vi "HEWH Channel Test Labels.vi"(0 "RunTime":bool) -> (3 "MW100 Channel Label":string[](array[string]), 4 "Agilent Cluster Array":T2[](array[typedef]), 6 "Channel List":string)   [LabVIEW 2016]
uses:
  Type Definitions/HEWH Channel Label.ctl
  Type Definitions/HEWH Agilent Cluster.ctl
  <vilib>/Utility/file.llb/Write To Spreadsheet File (string).vi
  <vilib>/Utility/file.llb/Read From Spreadsheet File (string).vi
panel:
  in  "Sensor 5":T1
  in  "Read TC Tree":bool
  out "Description":string="Thermocouple Setup"
  in  "Tab Control":enum32{"Page 1", "Page 2"}(tab)
  out "Agilent TC Locations":string[][](array[string])
  in  "Read":bool
  in  "Write":bool
  in  "Sensor 4":T1
  in  "Read None":bool
  in  "Sensor 3":T1
  in  "Read All":bool
  in  "Complete":bool
  in  "Panel 3":T1[][](array[typedef])=[[{"Label"="TC Cond1 - IN", "Chan"="301", "Rec"=TRUE}, {"Label"="TC Cond2", "Chan"="302", "Rec"=TRUE}, {"Label"="TC Cond3", "Chan"="303", "Rec"=TRUE}, {"Label"="TC Cond4", "Chan"="304", "Rec"=TRUE}, {"Label"="TC Cond5", "Chan"="305", "Rec"=TRUE}, {"Label"="TC Cond6", "Chan"="306", "Rec"=TRUE}], [{"Label"="TC Cond7", "Chan"="307", "Rec"=TRUE}, {"Label"="TC Cond8", "Chan"="308", "Rec"=TRUE}, {"Label"="TC Cond9", "Chan"="309", "Rec"=TRUE}, {"Label"="TC Cond10", "Chan"="310", "Rec"=TRUE}, {"Label"="TC Cond11", "Chan"="311", "Rec"=TRUE}, {"Label"="TC Cond12 - OUT", "Chan"="312", "Rec"=TRUE}], [{"Label"="TC Xtra 4", "Chan"="313", "Rec"=TRUE}, {"Label"="TC Xtra 5", "Chan"="314", "Rec"=TRUE}, {"Label"="TC Xtra 6", "Chan"="315", "Rec"=TRUE}, {"Label"="TC Xtra 7", "Chan"="316", "Rec"=TRUE}, {"Label"="TC Xtra 8", "Chan"="105", "Rec"=TRUE}, {"Label"="TC Xtra 9", "Chan"="106", "Rec"=TRUE}]]
  in  "Panel 2":T1[][](array[typedef])=[[{"Label"="TC Dry/W bulb 1", "Chan"="201", "Rec"=TRUE}, {"Label"="TC Dry/W bulb 2", "Chan"="202", "Rec"=TRUE}, {"Label"="TC Dry/W bulb 3", "Chan"="203", "Rec"=TRUE}, {"Label"="TC Dry/W bulb 4", "Chan"="204", "Rec"=TRUE}, {"Label"="TC Tsuction", "Chan"="205", "Rec"=TRUE}, {"Label"="TC Tdis", "Chan"="206", "Rec"=TRUE}], [{"Label"="TC Tret", "Chan"="207", "Rec"=TRUE}, {"Label"="TC Controls 1", "Chan"="208", "Rec"=TRUE}, {"Label"="TC Controls 2", "Chan"="209", "Rec"=TRUE}, {"Label"="TC Controls 3", "Chan"="210", "Rec"=TRUE}, {"Label"="TC Controls 4", "Chan"="211", "Rec"=TRUE}, {"Label"="TC Controls 5", "Chan"="212", "Rec"=TRUE}], [{"Label"="TC Shadow T1", "Chan"="213", "Rec"=TRUE}, {"Label"="TC Shadow T2", "Chan"="214", "Rec"=TRUE}, {"Label"="TC Shadow T3", "Chan"="215", "Rec"=TRUE}, {"Label"="TC Shadow T4", "Chan"="216", "Rec"=TRUE}, {"Label"="TC Shadow T5", "Chan"="107", "Rec"=TRUE}, {"Label"="TC Shadow T6", "Chan"="108", "Rec"=TRUE}]]
  in  "Panel 1":T1[][](array[typedef])=[[{"Label"="TC Tree 1 - TOP", "Chan"="", "Rec"=TRUE}, {"Label"="TC Tree 2", "Chan"="", "Rec"=TRUE}, {"Label"="TC Tree 3", "Chan"="", "Rec"=TRUE}, {"Label"="TC Tree 4", "Chan"="", "Rec"=TRUE}, {"Label"="TC Tree 5", "Chan"="", "Rec"=TRUE}, {"Label"="TC Tree 6 - BOT", "Chan"="", "Rec"=TRUE}], [{"Label"="TC Shell 1", "Chan"="", "Rec"=TRUE}, {"Label"="TC Shell 2", "Chan"="", "Rec"=TRUE}, {"Label"="TC Shell 3", "Chan"="", "Rec"=TRUE}, {"Label"="TC Shell 4", "Chan"="", "Rec"=TRUE}, {"Label"="TC Evap1 - IN", "Chan"="111", "Rec"=TRUE}, {"Label"="TC Evap2", "Chan"="112", "Rec"=TRUE}], [{"Label"="TC Evap3", "Chan"="113", "Rec"=TRUE}, {"Label"="TC Evap4", "Chan"="114", "Rec"=TRUE}, {"Label"="TC Evap5 - OUT", "Chan"="115", "Rec"=TRUE}, {"Label"="TC Xtra 1", "Chan"="116", "Rec"=TRUE}, {"Label"="TC Xtra 2", "Chan"="109", "Rec"=TRUE}, {"Label"="TC Xtra 3", "Chan"="1100", "Rec"=TRUE}]]
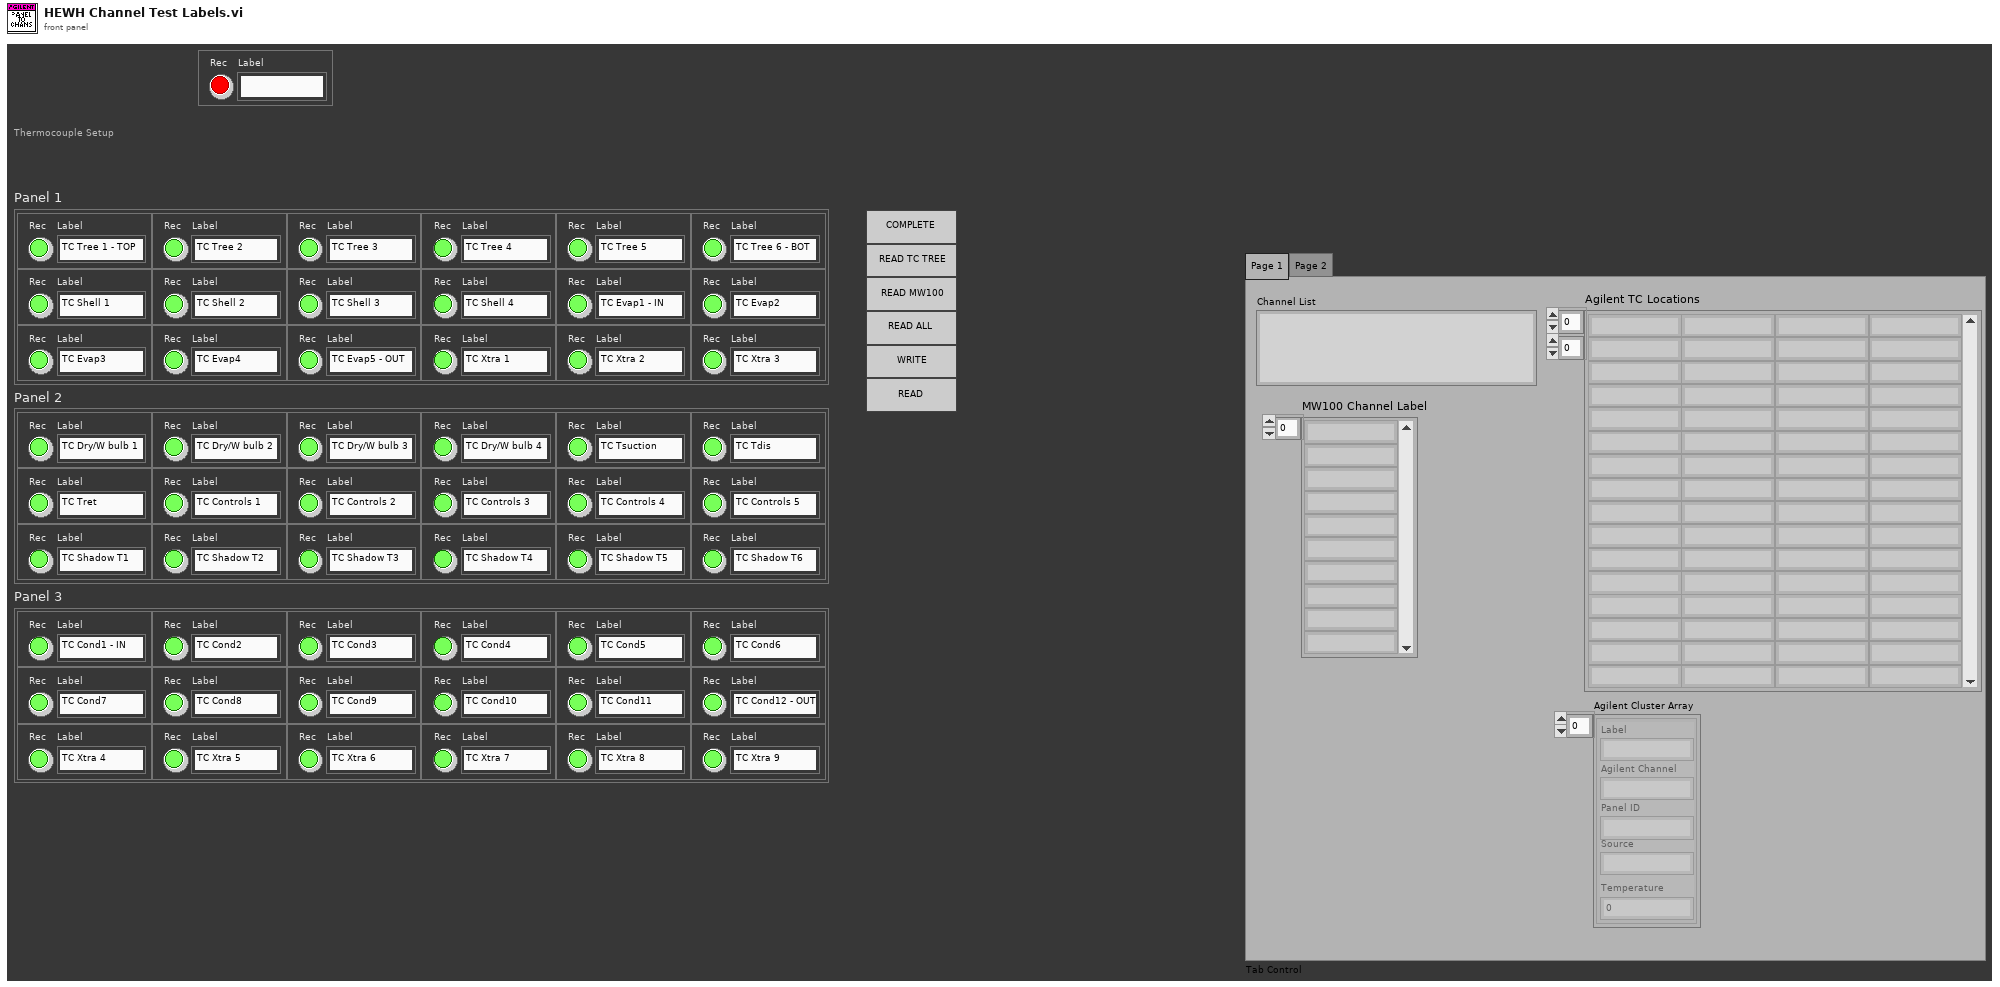
[diagram p1: front panel]
types:
  T1 = typedef "HEWH Channel Label.ctl" = cluster{"Label":string, "Chan":string, "Rec":bool}
  T2 = typedef "HEWH Agilent Cluster.ctl" = cluster{"Label":string, "Agilent Channel":string, "Panel ID":string, "Source":string, "Temperature":dbl}
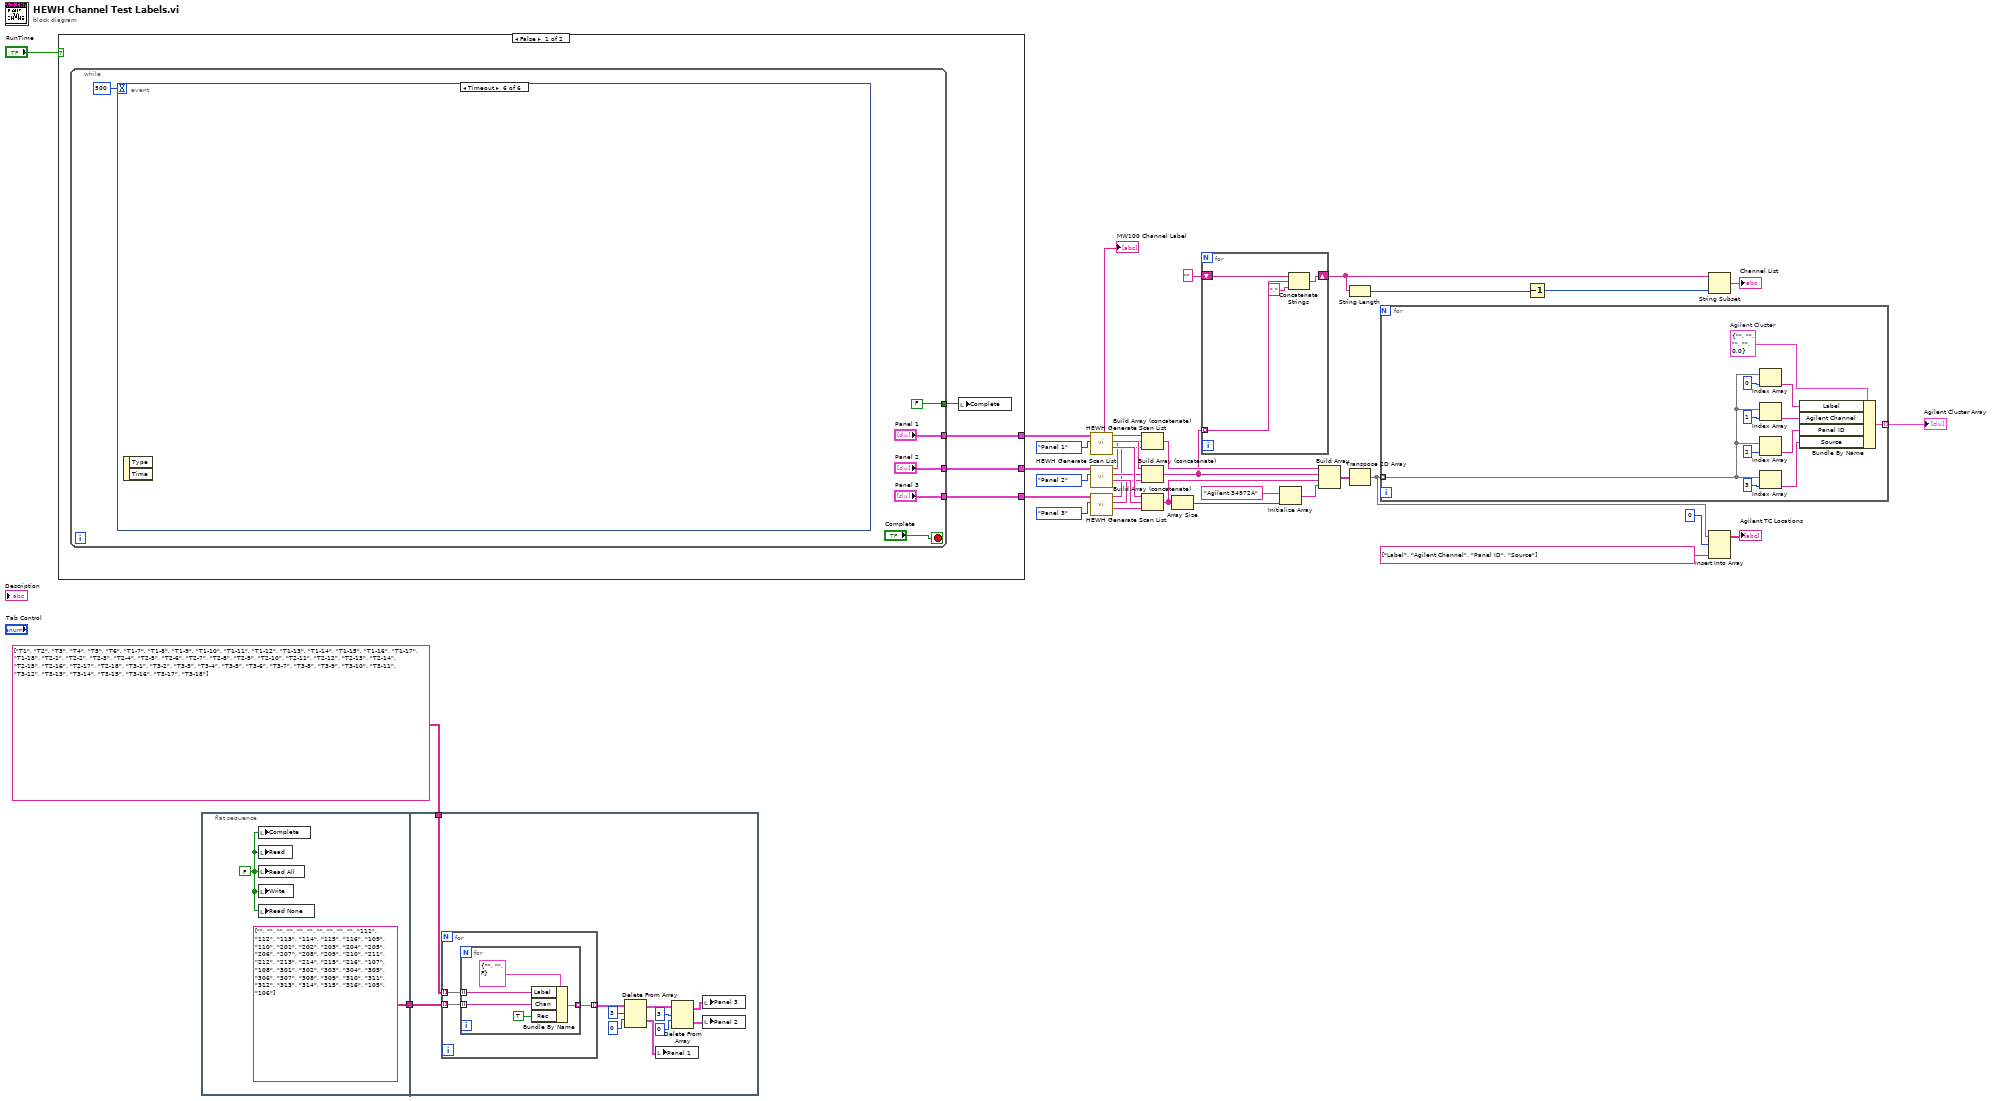
[diagram p0: block diagram]
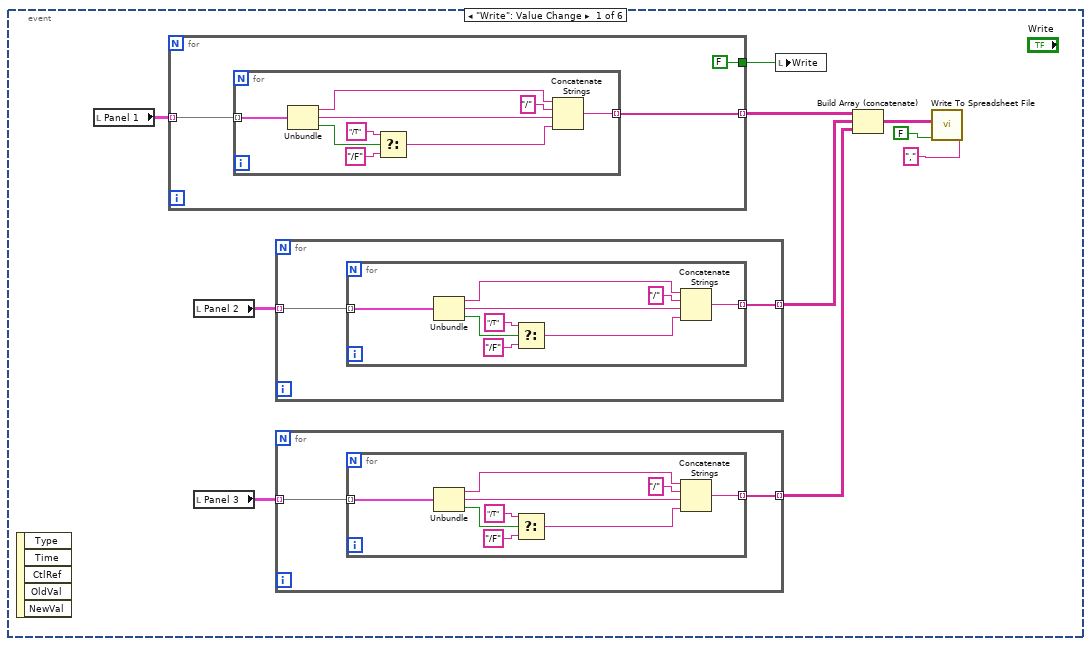
[diagram p2: hidden frame]
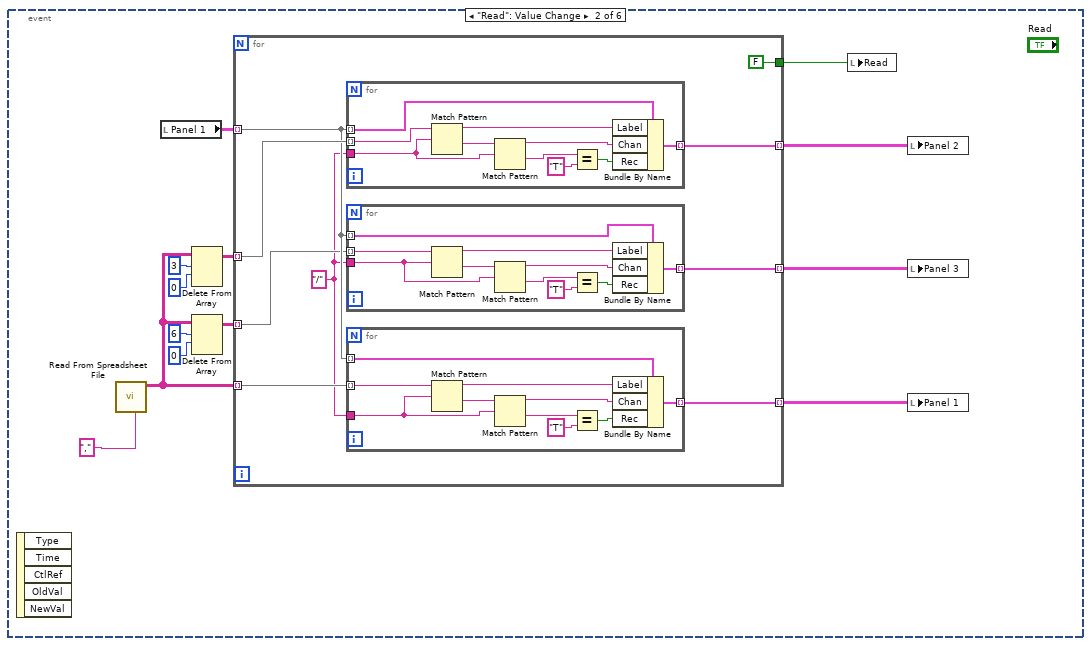
[diagram p3: hidden frame]
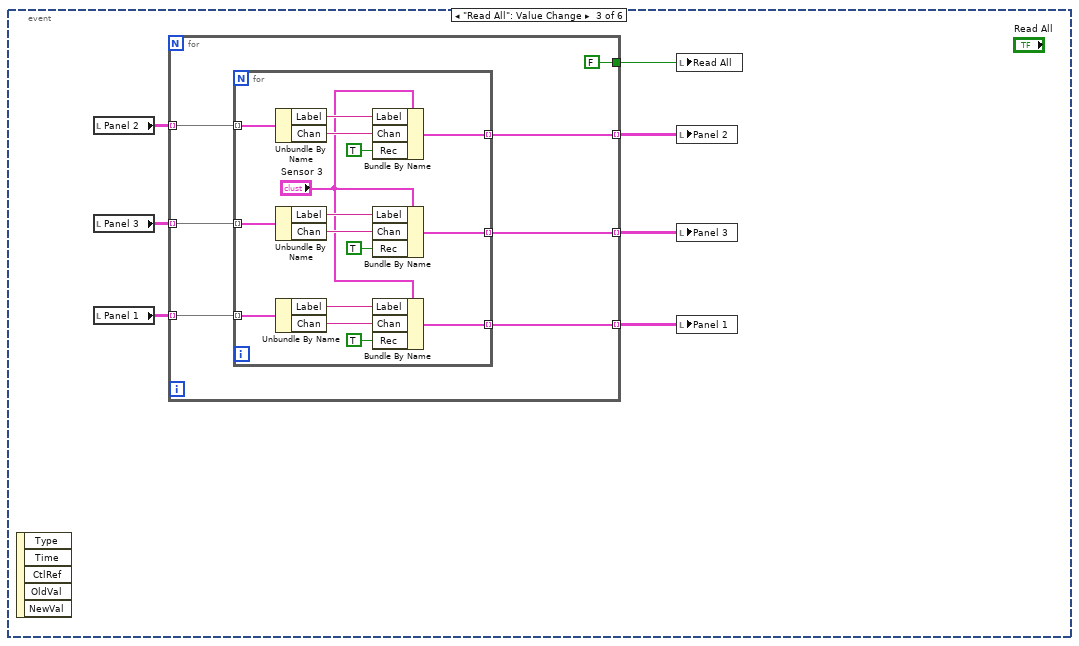
[diagram p4: hidden frame]
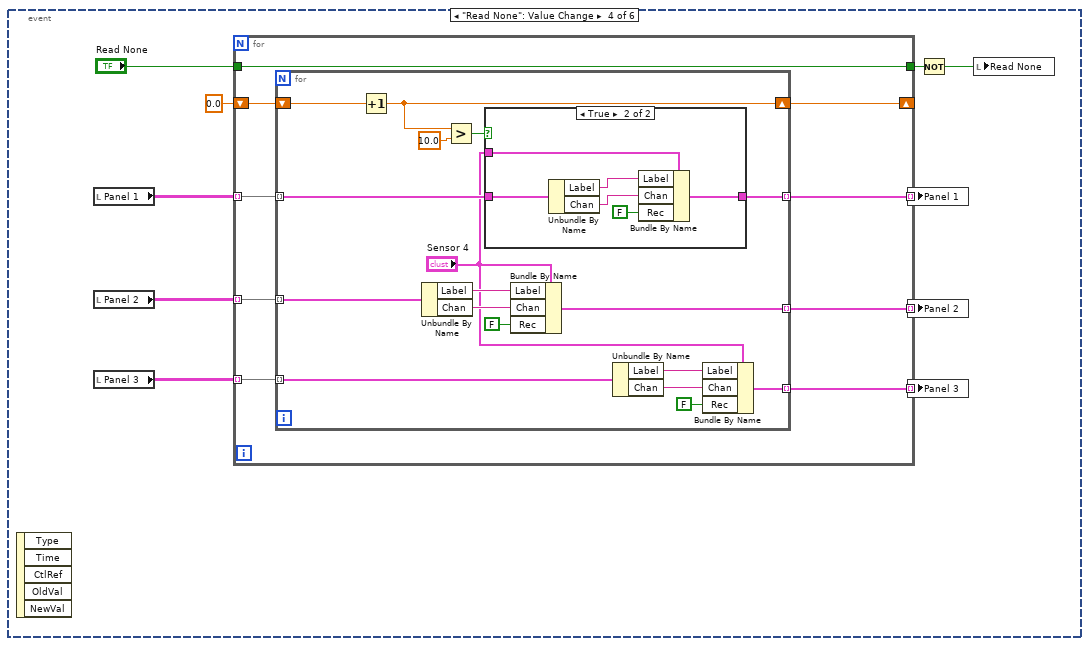
[diagram p5: hidden frame]
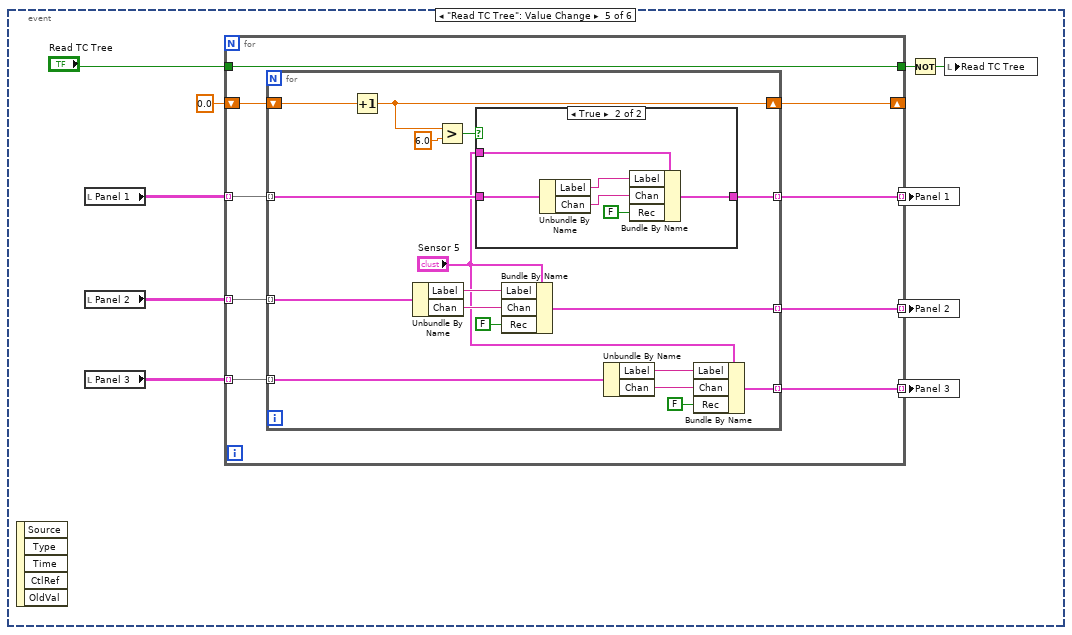
[diagram p7: hidden frame]
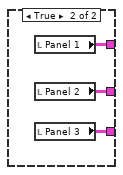
[diagram p9: hidden frame]
diagram:
  n1 = case shown="False" "RunTime" {
    tunnel: [w40 w261] -> w36
    tunnel: [w38 w260] -> w23
    tunnel: [w37 w259] -> w21
    frame False {
      n2 = while {
        tunnel: ["Panel 1"] -> w40
        tunnel: ["Panel 2"] -> w38
        tunnel: ["Panel 3"] -> w37
        tunnel: [FALSE ("Read None")] -> w39
        stop <- "Complete" stop-if-true
        n3 = event shown="[5] Timeout" {
          selector: _ -> [_ _ _ _ _ _]
          dyn-events: _ -> [_ _ _ _ _ _]
          timeout: 500 -> [_ _ _ _ _ _]
          event "Write": Value Change {
            n4 = event-data() -> ()  [unwired: 1 in, 5 out]
            n5 = local read "Panel 1"() -> (w55:T1[][])
            n6 = for {
              tunnel: w55 -> [w81] mode=indexing
              tunnel: [FALSE ("Read None")] -> w56
              tunnel: [w79] -> w51 mode=indexing
              n7 = for {
                tunnel: w81 -> [w90] mode=indexing
                tunnel: [w82] -> w79 mode=indexing
                n8 = Unbundle(w90) -> ("Label"=w89:string, "Chan"=w87:string, "Rec"=w84:bool)
                n9 = Select(t="/T" ("string"), s=w84, f="/F" ("string")) -> (s? t:f=w83:string)
                n10 = Concatenate Strings(w89, "/" ("string"), w87, w83) -> (w82:string)
              }
            }
            n11 = local read "Panel 2"() -> (w53:T1[][])
            n12 = local read "Panel 3"() -> (w52:T1[][])
            n13 = for {
              tunnel: w53 -> [w69] mode=indexing
              tunnel: [w68] -> w50 mode=indexing
              n14 = for {
                tunnel: w69 -> [w78] mode=indexing
                tunnel: [w70] -> w68 mode=indexing
                n15 = Unbundle(w78) -> ("Label"=w77:string, "Chan"=w75:string, "Rec"=w72:bool)
                n16 = Select(t="/T" ("string"), s=w72, f="/F" ("string")) -> (s? t:f=w71:string)
                n17 = Concatenate Strings(w77, "/" ("string"), w75, w71) -> (w70:string)
              }
            }
            n18 = for {
              tunnel: w52 -> [w58] mode=indexing
              tunnel: [w57] -> w49 mode=indexing
              n19 = for {
                tunnel: w58 -> [w67] mode=indexing
                tunnel: [w59] -> w57 mode=indexing
                n20 = Unbundle(w67) -> ("Label"=w66:string, "Chan"=w64:string, "Rec"=w61:bool)
                n21 = Select(t="/T" ("string"), s=w61, f="/F" ("string")) -> (s? t:f=w60:string)
                n22 = Concatenate Strings(w66, "/" ("string"), w64, w60) -> (w59:string)
              }
            }
            n23 = local write "Write"(w56) -> ()
            n24 = Build Array (concatenate)(w51, w50, w49) -> (w47:string[][])
            n25 = call-poly <vilib>:"Write To Spreadsheet File.vi"("delimiter (\\t)"="," ("delimiter (\\t)"), "append to file? (new file:F)"=FALSE ("Keep Refnum Open"), "2D data"=w47) -> ()  [unwired: 5 in, 1 out]
          }
          event "Read": Value Change {
            n26 = event-data() -> ()  [unwired: 1 in, 5 out]
            n27 = call-poly <vilib>:"Read From Spreadsheet File.vi"("delimiter (\\t)"="," ("delimiter (\\t)")) -> ("all rows"=w97:string[][])  [unwired: 6 in, 4 out]
            n28 = local read "Panel 1"() -> (w93:T1[][])
            n29 = Delete From Array(array=w97, length=3, index (row)=0) -> (array with subset deleted=w98:string[][])  [unwired: 1 in, 1 out]
            n30 = Delete From Array(array=w97, length=6, index (row)=0) -> (array with subset deleted=w99:string[][])  [unwired: 1 in, 1 out]
            n31 = for {
              tunnel: w93 -> [w107] mode=indexing
              tunnel: w97 -> [w112] mode=indexing
              tunnel: [w111] -> w96 mode=indexing
              tunnel: w98 -> [w110] mode=indexing
              tunnel: w99 -> [w106] mode=indexing
              tunnel: [w109] -> w95 mode=indexing
              tunnel: [w108] -> w94 mode=indexing
              tunnel: [FALSE ("Read")] -> w92
              w105 = "/" ("regular expression")
              n32 = for {
                tunnel: w107 -> [w131] mode=indexing
                tunnel: w110 -> [w132] mode=indexing
                tunnel: [w129] -> w109 mode=indexing
                tunnel: w105 -> [w123]
                n33 = Match Pattern(string=w132, regular expression=w123) -> (before substring=w130:string, after substring=w128:string)  [unwired: 1 in, 2 out]
                n34 = Match Pattern(string=w128, regular expression=w123) -> (before substring=w127:string, after substring=w126:string)  [unwired: 1 in, 2 out]
                n35 = Equal?(x=w126, y="T") -> (x = y?=w124:bool)
                n36 = Bundle By Name(cluster=w131, "Label"=w130, "Chan"=w127, "Rec"=w124) -> (w129:T1)
              }
              n37 = for {
                tunnel: w107 -> [w121] mode=indexing
                tunnel: w106 -> [w122] mode=indexing
                tunnel: [w119] -> w108 mode=indexing
                tunnel: w105 -> [w113]
                n38 = Match Pattern(string=w122, regular expression=w113) -> (before substring=w120:string, after substring=w118:string)  [unwired: 1 in, 2 out]
                n39 = Match Pattern(string=w118, regular expression=w113) -> (before substring=w117:string, after substring=w116:string)  [unwired: 1 in, 2 out]
                n40 = Equal?(x=w116, y="T") -> (x = y?=w114:bool)
                n41 = Bundle By Name(cluster=w121, "Label"=w120, "Chan"=w117, "Rec"=w114) -> (w119:T1)
              }
              n42 = for {
                tunnel: w107 -> [w141] mode=indexing
                tunnel: w112 -> [w142] mode=indexing
                tunnel: [w139] -> w111 mode=indexing
                tunnel: w105 -> [w133]
                n43 = Match Pattern(string=w142, regular expression=w133) -> (before substring=w140:string, after substring=w138:string)  [unwired: 1 in, 2 out]
                n44 = Match Pattern(string=w138, regular expression=w133) -> (before substring=w137:string, after substring=w136:string)  [unwired: 1 in, 2 out]
                n45 = Equal?(x=w136, y="T") -> (x = y?=w134:bool)
                n46 = Bundle By Name(cluster=w141, "Label"=w140, "Chan"=w137, "Rec"=w134) -> (w139:T1)
              }
            }
            n47 = local write "Read"(w92) -> ()
            n48 = local write "Panel 2"(w95) -> ()
            n49 = local write "Panel 3"(w94) -> ()
            n50 = local write "Panel 1"(w96) -> ()
          }
          event "Read All": Value Change {
            n51 = event-data() -> ()  [unwired: 1 in, 5 out]
            n52 = local read "Panel 2"() -> (w146:T1[][])
            n53 = local read "Panel 3"() -> (w145:T1[][])
            n54 = local read "Panel 1"() -> (w149:T1[][])
            n55 = for {
              tunnel: [w156] -> w148 mode=indexing
              tunnel: w149 -> [w155] mode=indexing
              tunnel: [w154] -> w147 mode=indexing
              tunnel: w146 -> [w153] mode=indexing
              tunnel: w145 -> [w152] mode=indexing
              tunnel: [w151] -> w144 mode=indexing
              tunnel: [FALSE ("Read None")] -> w143
              n56 = for {
                tunnel: [w172] -> w156 mode=indexing
                tunnel: w155 -> [w170] mode=indexing
                tunnel: [w164] -> w154 mode=indexing
                tunnel: w153 -> [w163] mode=indexing
                tunnel: w152 -> [w159] mode=indexing
                tunnel: [w158] -> w151 mode=indexing
                n57 = Unbundle By Name(w163) -> ("Label"=w166:string, "Chan"=w167:string)
                n58 = Unbundle By Name(w159) -> ("Label"=w161:string, "Chan"=w160:string)
                n59 = Unbundle By Name(w170) -> ("Label"=w169:string, "Chan"=w168:string)
                n60 = Bundle By Name(cluster="Sensor 3", "Label"=w166, "Chan"=w167, "Rec"=TRUE) -> (w164:T1)
                n61 = Bundle By Name(cluster="Sensor 3", "Label"=w161, "Chan"=w160, "Rec"=TRUE) -> (w158:T1)
                n62 = Bundle By Name(cluster="Sensor 3", "Label"=w169, "Chan"=w168, "Rec"=TRUE) -> (w172:T1)
              }
            }
            n63 = local write "Read All"(w143) -> ()
            n64 = local write "Panel 2"(w147) -> ()
            n65 = local write "Panel 3"(w144) -> ()
            n66 = local write "Panel 1"(w148) -> ()
          }
          event "Read None": Value Change {
            n67 = event-data() -> ()  [unwired: 1 in, 5 out]
            n68 = local read "Panel 1"() -> (w182:T1[][])
            n69 = local read "Panel 2"() -> (w179:T1[][])
            n70 = local read "Panel 3"() -> (w178:T1[][])
            n71 = for {
              tunnel: [w191] -> w181 mode=indexing
              tunnel: w182 -> [w190] mode=indexing
              tunnel: [w189] -> w180 mode=indexing
              tunnel: w179 -> [w188] mode=indexing
              tunnel: w178 -> [w187] mode=indexing
              tunnel: [w186] -> w177 mode=indexing
              tunnel: [w185] -> w175
              tunnel: "Read None" -> [w185]
              shift-right: [w183] -> _
              shift-left: 0.0 -> [w184]
              n72 = for {
                tunnel: [w208] -> w191 mode=indexing
                tunnel: w190 -> [w207] mode=indexing
                tunnel: [w203] -> w189 mode=indexing
                tunnel: w188 -> [w202] mode=indexing
                tunnel: w187 -> [w198] mode=indexing
                tunnel: [w197] -> w186 mode=indexing
                shift-right: [w194] -> w183
                shift-left: w184 -> [w195]
                n73 = Increment(x=w195) -> (x+1=w194:dbl)
                n74 = Unbundle By Name(w202) -> ("Label"=w205:string, "Chan"=w206:string)
                n75 = Greater?(x=w194, y=10.0) -> (0:w192:bool)
                n76 = case shown="True" w192 {
                  tunnel: [w209 w215] -> w208
                  tunnel: w207 -> [w209 w213]
                  tunnel: "Sensor 4" -> [_ w210]
                  frame False {
                  }
                  frame True {
                    n77 = Unbundle By Name(w213) -> ("Label"=w212:string, "Chan"=w211:string)
                    n78 = Bundle By Name(cluster=w210, "Label"=w212, "Chan"=w211, "Rec"=FALSE) -> (w215:T1)
                  }
                }
                n79 = Bundle By Name(cluster="Sensor 4", "Label"=w205, "Chan"=w206, "Rec"=FALSE) -> (w203:T1)
                n80 = Unbundle By Name(w198) -> ("Label"=w200:string, "Chan"=w199:string)
                n81 = Bundle By Name(cluster="Sensor 4", "Label"=w200, "Chan"=w199, "Rec"=FALSE) -> (w197:T1)
              }
            }
            n82 = local write "Panel 1"(w181) -> ()
            n83 = local write "Panel 2"(w180) -> ()
            n84 = local write "Panel 3"(w177) -> ()
            n85 = Not(x=w175) -> (.not. x?=w176:bool)
            n86 = local write "Read None"(w176) -> ()
          }
          event "Read TC Tree": Value Change {
            n87 = event-data() -> ()  [unwired: 1 in, 5 out]
            n88 = local read "Panel 1"() -> (w225:T1[][])
            n89 = local read "Panel 2"() -> (w222:T1[][])
            n90 = local read "Panel 3"() -> (w221:T1[][])
            n91 = for {
              tunnel: [w234] -> w224 mode=indexing
              tunnel: w225 -> [w233] mode=indexing
              tunnel: [w232] -> w223 mode=indexing
              tunnel: w222 -> [w231] mode=indexing
              tunnel: w221 -> [w230] mode=indexing
              tunnel: [w229] -> w220 mode=indexing
              tunnel: [w228] -> w219
              tunnel: "Read TC Tree" -> [w228]
              shift-right: [w226] -> _
              shift-left: 0.0 -> [w227]
              n92 = for {
                tunnel: [w251] -> w234 mode=indexing
                tunnel: w233 -> [w250] mode=indexing
                tunnel: [w246] -> w232 mode=indexing
                tunnel: w231 -> [w245] mode=indexing
                tunnel: w230 -> [w241] mode=indexing
                tunnel: [w240] -> w229 mode=indexing
                shift-right: [w237] -> w226
                shift-left: w227 -> [w238]
                n93 = Increment(x=w238) -> (x+1=w237:dbl)
                n94 = Unbundle By Name(w245) -> ("Label"=w248:string, "Chan"=w249:string)
                n95 = Greater?(x=w237, y=6.0) -> (0:w235:bool)
                n96 = case shown="True" w235 {
                  tunnel: [w252 w258] -> w251
                  tunnel: w250 -> [w252 w256]
                  tunnel: "Sensor 5" -> [_ w253]
                  frame False {
                  }
                  frame True {
                    n97 = Unbundle By Name(w256) -> ("Label"=w255:string, "Chan"=w254:string)
                    n98 = Bundle By Name(cluster=w253, "Label"=w255, "Chan"=w254, "Rec"=FALSE) -> (w258:T1)
                  }
                }
                n99 = Bundle By Name(cluster="Sensor 5", "Label"=w248, "Chan"=w249, "Rec"=FALSE) -> (w246:T1)
                n100 = Unbundle By Name(w241) -> ("Label"=w243:string, "Chan"=w242:string)
                n101 = Bundle By Name(cluster="Sensor 5", "Label"=w243, "Chan"=w242, "Rec"=FALSE) -> (w240:T1)
              }
            }
            n102 = local write "Panel 1"(w224) -> ()
            n103 = local write "Panel 2"(w223) -> ()
            n104 = local write "Panel 3"(w220) -> ()
            n105 = Not(x=w219) -> (.not. x?=w216:bool)
            n106 = local write "Read TC Tree"(w216) -> ()
          }
          event Timeout {
            n107 = event-data() -> ()  [unwired: 1 in, 2 out]
          }
        }
      }
      n108 = local write "Complete"(w39) -> ()
    }
    frame True {
      n109 = local read "Panel 1"() -> (w261:T1[][])
      n110 = local read "Panel 2"() -> (w260:T1[][])
      n111 = local read "Panel 3"() -> (w259:T1[][])
    }
  }
  n112 = flat-sequence {
    tunnel: [string[][] [["", "", "", "", "", ""], ["", "", "", "", "111", "112"], ["113", "114", "115", "116", "109", "110"], ["201", "202", "203", "204", "205", "206"], ["207", "208", "209", "210", "211", "212"], ["213", "214", "215", "216", "107", "108"], ["301", "302", "303", "304", "305", "306"], ["307", "308", "309", "310", "311", "312"], ["313", "314", "315", "316", "105", "106"]] ("transposed array")] -> w13
    tunnel: w13 -> [w265]
    tunnel: string[][] [["T1", "T2", "T3", "T4", "T5", "T6"], ["T1-7", "T1-8", "T1-9", "T1-10", "T1-11", "T1-12"], ["T1-13", "T1-14", "T1-15", "T1-16", "T1-17", "T1-18"], ["T2-1", "T2-2", "T2-3", "T2-4", "T2-5", "T2-6"], ["T2-7", "T2-8", "T2-9", "T2-10", "T2-11", "T2-12"], ["T2-13", "T2-14", "T2-15", "T2-16", "T2-17", "T2-18"], ["T3-1", "T3-2", "T3-3", "T3-4", "T3-5", "T3-6"], ["T3-7", "T3-8", "T3-9", "T3-10", "T3-11", "T3-12"], ["T3-13", "T3-14", "T3-15", "T3-16", "T3-17", "T3-18"]] ("Array") -> [w264]
    frame #0 {
      w262 = FALSE ("Read None")
      n113 = local write "Complete"(w262) -> ()
      n114 = local write "Read"(w262) -> ()
      n115 = local write "Read All"(w262) -> ()
      n116 = local write "Write"(w262) -> ()
      n117 = local write "Read None"(w262) -> ()
    }
    frame #1 {
      n118 = for {
        tunnel: [w277] -> w274 mode=indexing
        tunnel: w264 -> [w276] mode=indexing
        tunnel: w265 -> [w275] mode=indexing
        n119 = for {
          tunnel: [w282] -> w277 mode=indexing
          tunnel: w276 -> [w281] mode=indexing
          tunnel: w275 -> [w280] mode=indexing
          n120 = Bundle By Name(cluster=T1 {"Label"="", "Chan"="", "Rec"=FALSE} ("Sensor 2"), "Label"=w281, "Chan"=w280, "Rec"=TRUE) -> (w282:T1)
        }
      }
      n121 = Delete From Array(array=w274, length=3, index (row)=0) -> (deleted portion=w268:T1[][], array with subset deleted=w269:T1[][])  [unwired: 1 in]
      n122 = local write "Panel 1"(w268) -> ()
      n123 = Delete From Array(array=w269, length=3, index (row)=0) -> (deleted portion=w267:T1[][], array with subset deleted=w266:T1[][])  [unwired: 1 in]
      n124 = local write "Panel 3"(w266) -> ()
      n125 = local write "Panel 2"(w267) -> ()
    }
  }
  n126 = call "HEWH Generate Scan List.vi"(10:"Panel"=enum16{"Panel 1", "Panel 2", "Panel 3"}."Panel 1" ("Panel"), 11:"Panel"=w36) -> ("Panel List"=w28:string[], "Channel Number"=w34:string[], "Channel Label"=w35:string[], "MW100 Channel Label"=→"MW100 Channel Label":string[])  [unwired: 6 in]
  n127 = call "HEWH Generate Scan List.vi"(10:"Panel"=enum16{"Panel 1", "Panel 2", "Panel 3"}."Panel 2" ("Panel"), 11:"Panel"=w23) -> ("Panel List"=w19:string[], "Channel Number"=w17:string[], "Channel Label"=w18:string[])  [unwired: 6 in, 1 out]
  n128 = call "HEWH Generate Scan List.vi"(10:"Panel"=enum16{"Panel 1", "Panel 2", "Panel 3"}."Panel 3" ("Panel"), 11:"Panel"=w21) -> ("Panel List"=w16:string[], "Channel Number"=w14:string[], "Channel Label"=w15:string[])  [unwired: 6 in, 1 out]
  n129 = Build Array (concatenate)(w35, w18, w15) -> (w27:string[])
  n130 = Build Array (concatenate)(w34, w17, w14) -> (w26:string[])
  n131 = Build Array (concatenate)(w28, w19, w16) -> (w6:string[])
  n132 = Array Size(array=w6) -> (size(s)=w5:i32)
  n133 = for {
    tunnel: w26 -> [w285] mode=indexing
    shift-right: [w284] -> w32
    shift-left: "" -> [w283]
    n134 = Concatenate Strings(w283, w285, "," ("string")) -> (w284:string)
  }
  n135 = Initialize Array("Agilent 34972A", w5) -> (w4:string[])
  n136 = Build Array(w27, w26, w6, w4) -> (w25:string[][])
  n137 = String Length(string=w32) -> (length=w30:i32)
  n138 = Transpose 2D Array(2D array=w25) -> (transposed array=w3:string[][])
  n139 = for {
    tunnel: w3 -> [w297] mode=indexing
    tunnel: [w288] -> w2 mode=indexing
    w287 = T2 {"Label"="", "Agilent Channel"="", "Panel ID"="", "Source"="", "Temperature"=0.0}  # Agilent Cluster
    n140 = Index Array(array=w297, index=0) -> (element=w292:string)
    n141 = Index Array(array=w297, index=1) -> (element=w291:string)
    n142 = Index Array(array=w297, index=2) -> (element=w290:string)
    n143 = Index Array(array=w297, index=3) -> (element=w289:string)
    n144 = Bundle By Name(cluster=w287, "Label"=w292, "Agilent Channel"=w291, "Panel ID"=w290, "Source"=w289) -> (w288:T2)
  }
  "Agilent Cluster Array" <- w2
  n145 = Decrement(x=w30) -> (x-1=w31:i32)
  n146 = String Subset(string=w32, length (rest)=w31) -> (substring=→"Channel List":string)  [unwired: 1 in]
  n147 = Insert Into Array(array=w3, index (row)=0, new element=string[] ["Label", "Agilent Channel", "Panel ID", "Source"] ("element")) -> (→"Agilent TC Locations":string[][])  [unwired: 1 in]
